vi "ThermalDiffusivity.vi"() -> ()   [LabVIEW 2014]
uses:
  Typedef_FindPortActions.ctl
  Typedef_TeachLabArduinos.ctl
  Typedef_DataLogger_Actions.ctl
  <vilib>/Utility/file.llb/Write To Spreadsheet File (DBL).vi
panel:
  out "Internal Temp vs Time":cluster{dbl[], dbl[]}(graph)
  out "External Temp":dbl format="%.2f"
  in  "Time Step (ms)":i32=500 min=5 max=5000 step=1
  out "Internal Temp":dbl format="%.2f"
  out "External Temp vs Time":cluster{dbl[], dbl[]}(graph)
  out "Elapsed Time (s)":dbl format="%.1f"
  in  "Filename Header":string="Data"
  in  "Maximum Log Time (s)":dbl=600.0 format="%#_6f"
  out "Status":enum16{"Logging", "Stopped"}(ring)=enum."Stopped"
  in  "Logging":cluster{"Start":bool, "Stop":bool}
  out "Last Save's Filename":string
  in  "Save Data":bool
  in  "Reset Graph":bool
  out "Error Out":errorcluster
  in  "Exit Program":bool
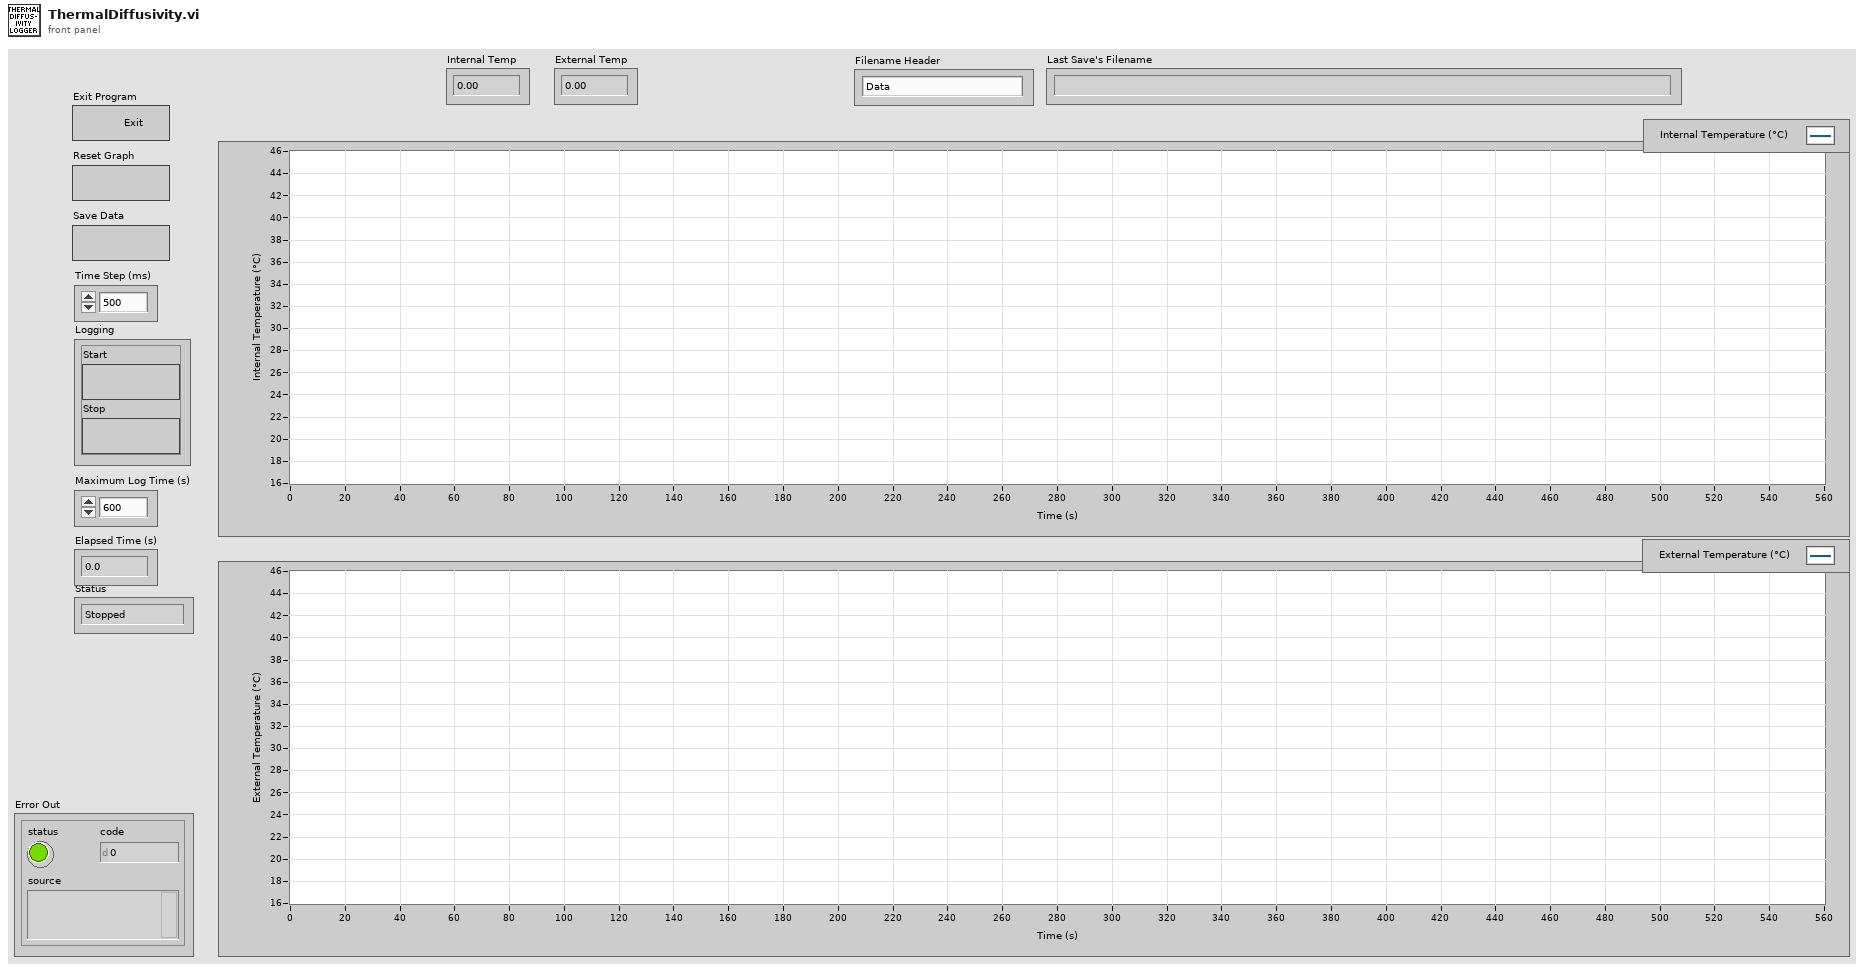
[diagram p1: front panel]
types:
  T1 = typedef "Typedef_FindPortActions.ctl" = enum16{"Reset List", "Find arduinos", "Get COM Port"}
  T2 = typedef "Typedef_TeachLabArduinos.ctl" = enum16{"FH", "AL", "CO", "TD"}
  T3 = typedef "Typedef_DataLogger_Actions.ctl" = enum16{"Connect", "Disconnect", "Get Reading", "Set Offset", "Get Offset", "Set Time Step", "Get Time Step", "Save Settings", "Disable Readings", "Enable Readings"}
  T4 = cluster{cluster{dbl[], dbl[]}, cluster{dbl[], dbl[]}}
  T5 = cluster{"Internal Temp":dbl, "External Temp":dbl}
  T6 = cluster{"Internal Temp vs Time In":cluster{"Array":dbl[], "Array":dbl[]}, "External Temp vs Time In":cluster{"Array":dbl[], "Array":dbl[]}}
  T7 = enum32{"invalid app kind", "Development System", "Run Time System", "Student Edition", "Embedded LabVIEW", "Evaluation", "Custom"}
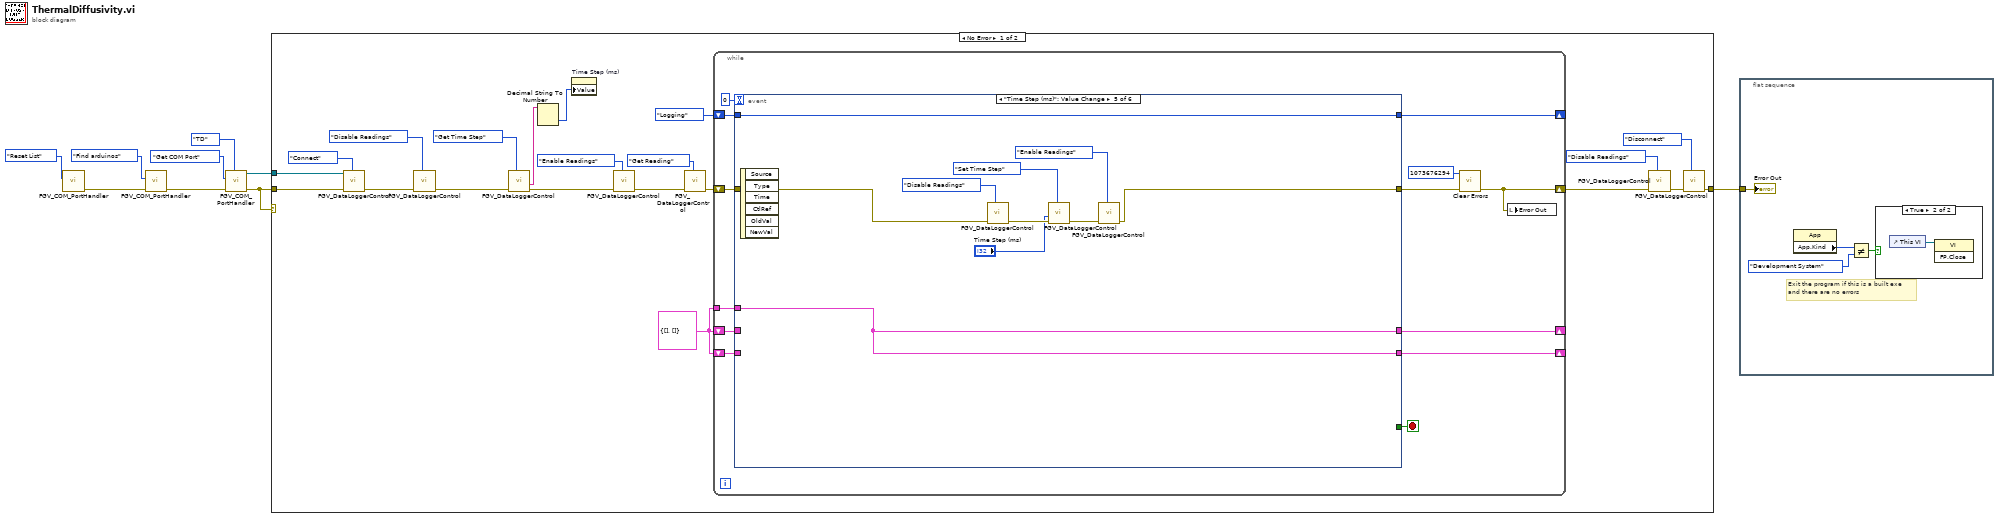
[diagram p0: block diagram]
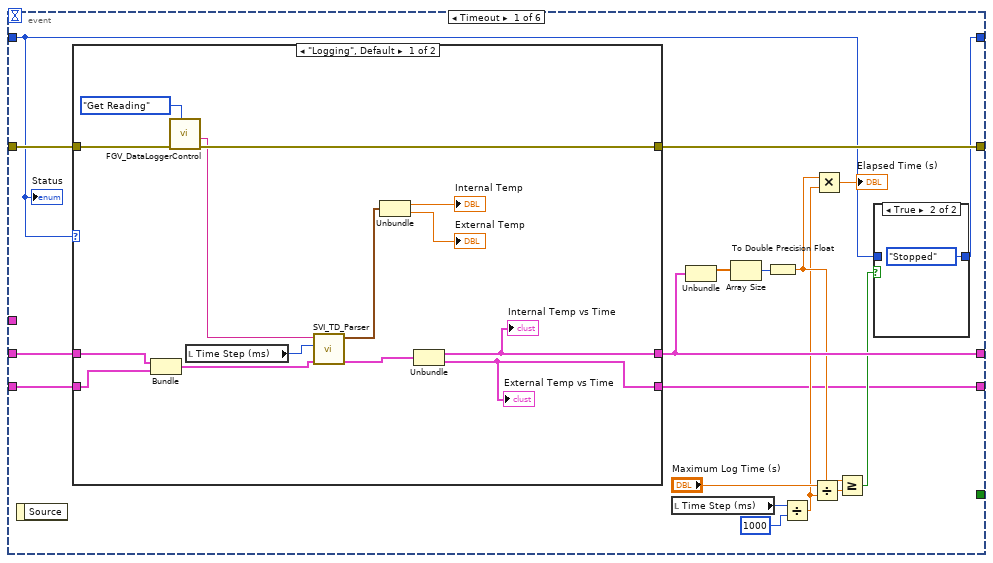
[diagram p3: hidden frame]
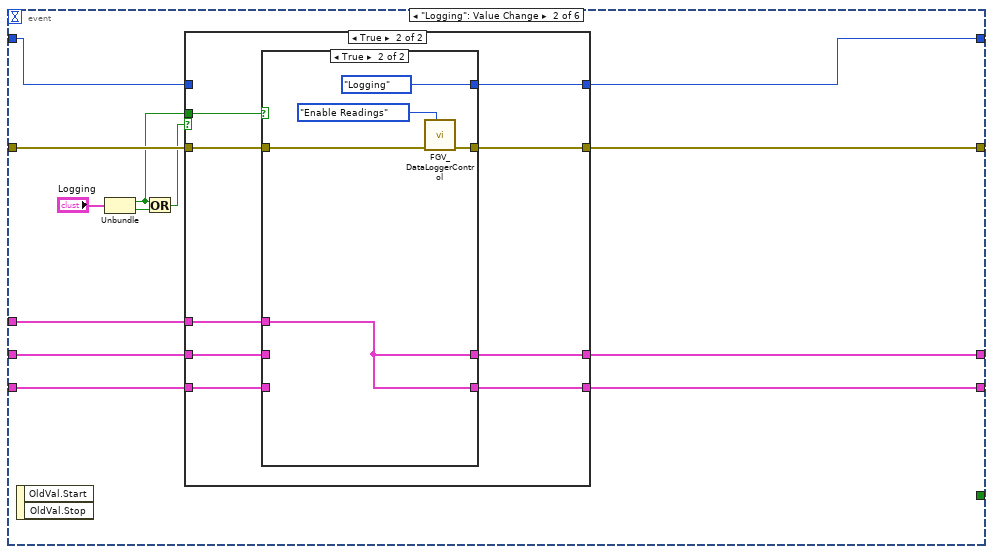
[diagram p6: hidden frame]
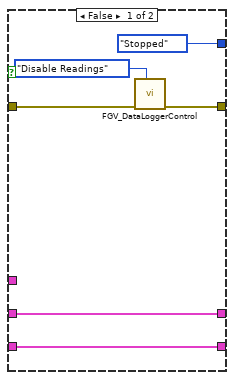
[diagram p8: hidden frame]
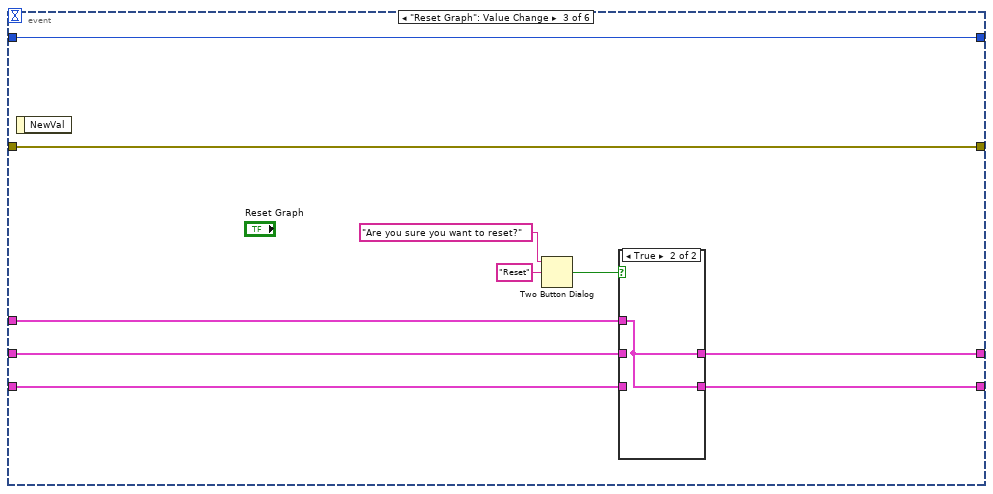
[diagram p9: hidden frame]
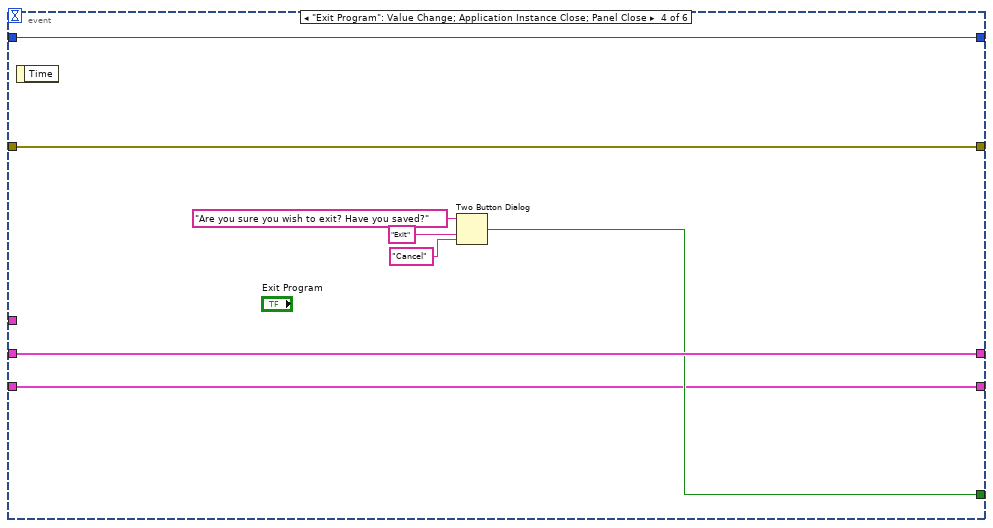
[diagram p11: hidden frame]
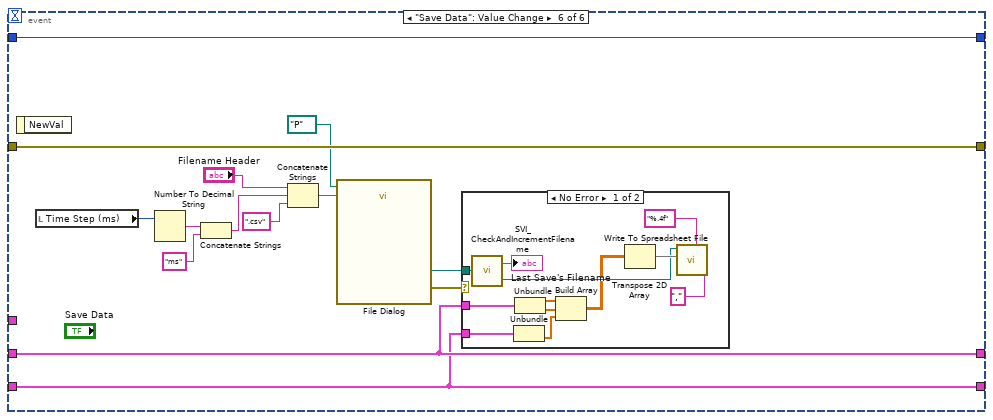
[diagram p12: hidden frame]
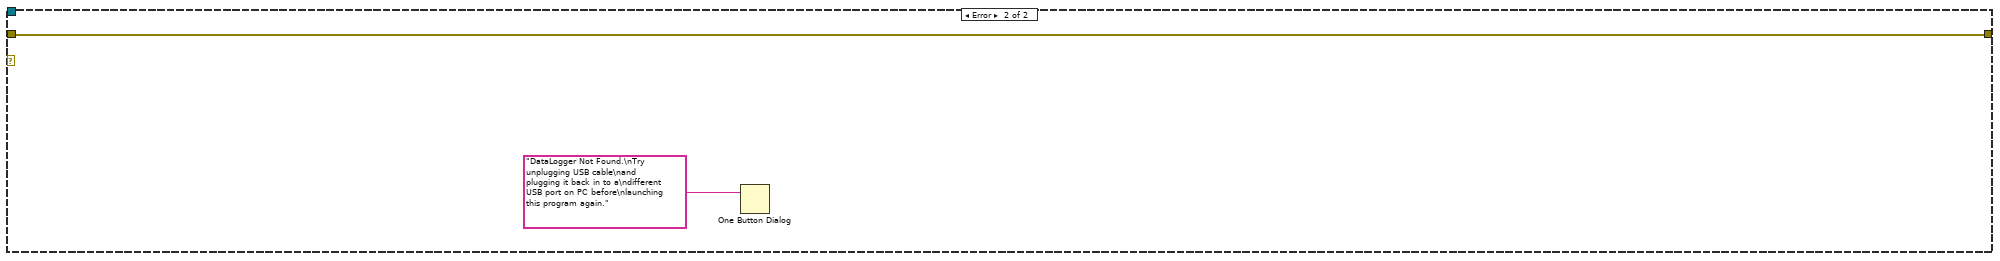
[diagram p14: hidden frame]
diagram:
  n1 = call "FGV_COM_PortHandler.vi"("Action"=Typedef_FindPortActions."Reset List") -> ("Error Out"=w5:errorcluster)  [unwired: 5 in, 2 out]
  n2 = call "FGV_COM_PortHandler.vi"("Error In"=w5, "Action"=Typedef_FindPortActions."Find arduinos") -> ("Error Out"=w9:errorcluster)  [unwired: 4 in, 2 out]
  n3 = call "FGV_COM_PortHandler.vi"("Device"=Typedef_TeachLabArduinos."TD", "Error In"=w9, "Action"=Typedef_FindPortActions."Get COM Port") -> ("Error Out"=w2:errorcluster, "COM Port"=w3:refnum<visa-resource-name>)  [unwired: 3 in, 1 out]
  n4 = case shown="No Error" w2 {
    tunnel: w2 -> [w29 w176]
    tunnel: w3 -> [w28 _]
    tunnel: [w25 w176] -> w1
    frame No Error {
      w10 = cluster{dbl[], dbl[]} {[], []}
      n5 = call "FGV_DataLoggerControl.vi"("Actions"=Typedef_DataLogger_Actions."Connect", "Error In"=w29, "VISA Refnum in"=w28) -> ("Error Out"=w21:errorcluster)  [unwired: 6 in, 2 out]
      n6 = call "FGV_DataLoggerControl.vi"("Actions"=Typedef_DataLogger_Actions."Disable Readings", "Error In"=w21) -> ("Error Out"=w20:errorcluster)  [unwired: 7 in, 2 out]
      n7 = call "FGV_DataLoggerControl.vi"("Actions"=Typedef_DataLogger_Actions."Get Time Step", "Error In"=w20) -> ("Error Out"=w18:errorcluster, "read buffer"=w24:string)  [unwired: 7 in, 1 out]
      n8 = Decimal String To Number(string=w24) -> (number=w23:i32)  [unwired: 2 in, 1 out]
      n9 = property on="Time Step (ms)" class="DigNum (strict)"("Value"=w23) -> ()  [unwired: 2 in, 2 out]
      n10 = call "FGV_DataLoggerControl.vi"("Actions"=Typedef_DataLogger_Actions."Enable Readings", "Error In"=w18) -> ("Error Out"=w11:errorcluster)  [unwired: 7 in, 2 out]
      n11 = call "FGV_DataLoggerControl.vi"("Actions"=Typedef_DataLogger_Actions."Get Reading", "Error In"=w11) -> ("Error Out"=w12:errorcluster)  [unwired: 7 in, 2 out]
      n12 = while {
        shift-right: [w40] -> _
        shift-left: w10 -> [w39]
        tunnel: w10 -> [w38]
        shift-right: [w36] -> _
        shift-left: enum16{"Logging", "Stopped"}."Logging" ("Status") -> [w37]
        shift-right: [w34] -> w16
        shift-left: w12 -> [w43]
        shift-right: [w31] -> _
        shift-left: w10 -> [w32]
        stop <- w42 stop-if-true
        n13 = event shown="[4] \"Time Step (ms)\": Value Change" {
          selector: _ -> [_ _ _ _ _ _]
          dyn-events: _ -> [_ _ _ _ _ _]
          timeout: 0 -> [_ _ _ _ _ _]
          tunnel: w43 -> [w61 w91 w127 w137 w142 w162]
          tunnel: [w60 w90 w127 w137 w143 w162] -> w33
          tunnel: [_ _ _ w133 _ _] -> w42
          tunnel: [w57 w84 w121 w138 w140 w150] -> w40
          tunnel: w39 -> [w59 w85 w119 w138 _ w150]
          tunnel: w38 -> [_ w83 w122 _ w140 _]
          tunnel: [w50 w93 w126 w132 w141 w154] -> w36
          tunnel: w37 -> [w49 w92 w126 w132 w141 w154]
          tunnel: w32 -> [w45 w81 w118 w131 _ w149]
          tunnel: [w44 w82 w120 w131 w140 w149] -> w31
          event Timeout {
            n14 = event-data() -> ()  [unwired: 1 in, 1 out]
            n15 = case shown="\"Logging\", Default" w49 {
              tunnel: w61 -> [w77 w79]
              tunnel: [w76 w79] -> w60
              tunnel: [w66 w80] -> w57
              tunnel: w59 -> [w71 w80]
              tunnel: w45 -> [w70 w78]
              tunnel: [w65 w78] -> w44
              frame "Logging", Default {
                n16 = Bundle(w71, w70) -> (w72:T4)  [unwired: 1 in]
                n17 = call "FGV_DataLoggerControl.vi"("Actions"=Typedef_DataLogger_Actions."Get Reading", "Error In"=w77) -> ("Error Out"=w76:errorcluster, "read buffer"=w74:string)  [unwired: 7 in, 1 out]
                n18 = local read "Time Step (ms)"() -> (w68:i32)
                n19 = call "SVI_TD_Parser.vi"("read buffer"=w74, "Time Step (ms)"=w68, "In"=w72) -> ("Current Values"=w67:T5, "Out"=w73:T6)  [unwired: 4 in]
                n20 = Unbundle(w67) -> ("Internal Temp"=→"Internal Temp":dbl, "External Temp"=→"External Temp":dbl)
                n21 = Unbundle(w73) -> ("Internal Temp vs Time In"=w66:cluster{"Array":dbl[], "Array":dbl[]}, "External Temp vs Time In"=w65:cluster{"Array":dbl[], "Array":dbl[]})
                "External Temp vs Time" <- w65
                "Internal Temp vs Time" <- w66
              }
              frame "Stopped" {
              }
            }
            n22 = local read "Time Step (ms)"() -> (w56:i32)
            n23 = Unbundle(w57) -> ("Array"=w58:dbl[])  [unwired: 1 out]
            n24 = Array Size(array=w58) -> (size(s)=w52:i32)
            n25 = To Double Precision Float(number=w52) -> (double precision float=w48:dbl)
            n26 = Divide(x=w56, y=1000) -> (x/y=w47:dbl)
            n27 = Divide(x="Maximum Log Time (s)", y=w47) -> (x/y=w53:dbl)
            n28 = Multiply(x=w48, y=w47) -> (x*y=→"Elapsed Time (s)":dbl)
            n29 = Greater Or Equal?(x=w48, y=w53) -> (x >= y?=w51:bool)
            n30 = case shown="True" w51 {
              tunnel: [w62 enum16{"Logging", "Stopped"}."Stopped" ("Status")] -> w50
              tunnel: w49 -> [w62 _]
              frame False {
              }
              frame True {
              }
            }
            "Status" <- w49
          }
          event "Logging": Value Change {
            n31 = event-data() -> ()  [unwired: 1 in, 2 out]
            n32 = Unbundle("Logging") -> ("Start"=w86:bool, "Stop"=w88:bool)
            n33 = Or(x=w86, y=w88) -> (x .or. y?=w87:bool)
            n34 = case shown="True" w87 {
              tunnel: [w97 w106] -> w93
              tunnel: w92 -> [w97 _]
              tunnel: w91 -> [w96 w105]
              tunnel: [w96 w104] -> w90
              tunnel: w86 -> [_ w103]
              tunnel: w85 -> [w95 w102]
              tunnel: [w95 w101] -> w84
              tunnel: w83 -> [_ w100]
              tunnel: [w94 w99] -> w82
              tunnel: w81 -> [w94 w98]
              frame False {
              }
              frame True {
                n35 = case shown="True" w103 {
                  tunnel: [enum16{"Logging", "Stopped"}."Stopped" ("Status") enum16{"Logging", "Stopped"}."Logging" ("Status")] -> w106
                  tunnel: w105 -> [w109 w115]
                  tunnel: [w110 w114] -> w104
                  tunnel: w102 -> [w108 _]
                  tunnel: [w108 w113] -> w101
                  tunnel: w100 -> [_ w113]
                  tunnel: [w107 w113] -> w99
                  tunnel: w98 -> [w107 _]
                  frame False {
                    n36 = call "FGV_DataLoggerControl.vi"("Actions"=Typedef_DataLogger_Actions."Disable Readings", "Error In"=w109) -> ("Error Out"=w110:errorcluster)  [unwired: 7 in, 2 out]
                  }
                  frame True {
                    n37 = call "FGV_DataLoggerControl.vi"("Actions"=Typedef_DataLogger_Actions."Enable Readings", "Error In"=w115) -> ("Error Out"=w114:errorcluster)  [unwired: 7 in, 2 out]
                  }
                }
              }
            }
          }
          event "Reset Graph": Value Change {
            n38 = event-data() -> ()  [unwired: 1 in, 1 out]
            n39 = Two Button Dialog(message="Are you sure you want to reset?", 2:"Reset" ("T button name (\"OK\")")) -> (T button?=w123:bool)  [unwired: 1 in]
            n40 = case shown="True" w123 {
              tunnel: w122 -> [_ w130]
              tunnel: [w129 w130] -> w121
              tunnel: [w128 w130] -> w120
              tunnel: w119 -> [w129 _]
              tunnel: w118 -> [w128 _]
              frame False {
              }
              frame True {
              }
            }
          }
          event "Exit Program": Value Change; Application Instance Close; Panel Close {
            n41 = event-data() -> ()  [unwired: 1 in, 1 out]
            n42 = Two Button Dialog(message="Are you sure you wish to exit? Have you saved?", 1:"Cancel" ("F button name (\"Cancel\")"), 2:"Exit" ("T button name (\"OK\")")) -> (T button?=w133:bool)
          }
          event "Time Step (ms)": Value Change {
            n43 = event-data() -> ()  [unwired: 1 in, 6 out]
            n44 = call "FGV_DataLoggerControl.vi"("Actions"=Typedef_DataLogger_Actions."Disable Readings", "Error In"=w142) -> ("Error Out"=w146:errorcluster)  [unwired: 7 in, 2 out]
            n45 = call "FGV_DataLoggerControl.vi"("Actions"=Typedef_DataLogger_Actions."Set Time Step", "Error In"=w146, "Value"="Time Step (ms)") -> ("Error Out"=w144:errorcluster)  [unwired: 6 in, 2 out]
            n46 = call "FGV_DataLoggerControl.vi"("Actions"=Typedef_DataLogger_Actions."Enable Readings", "Error In"=w144) -> ("Error Out"=w143:errorcluster)  [unwired: 7 in, 2 out]
          }
          event "Save Data": Value Change {
            n47 = event-data() -> ()  [unwired: 1 in, 1 out]
            n48 = local read "Time Step (ms)"() -> (w155:i32)
            n49 = Number To Decimal String(number=w155) -> (decimal integer string=w156:string)  [unwired: 1 in]
            n50 = Concatenate Strings(w156, "ms" ("string")) -> (w158:string)
            n51 = Concatenate Strings("Filename Header", w158, ".csv" ("default name")) -> (w160:string)
            n52 = call "File Dialog"("start path"=path "P:/", "default name"=w160) -> ("selected path"=w161:path, "error out"=w151:errorcluster)  [unwired: 10 in, 2 out]
            n53 = case shown="No Error" w151 {
              tunnel: w161 -> [w171 _]
              tunnel: w150 -> [w165 _]
              tunnel: w149 -> [w164 _]
              frame No Error {
                n54 = call "SVI_CheckAndIncrementFilename.vi"("selected path"=w171) -> ("Filename"=→"Last Save's Filename":string, "File Path"=w168:path)
                n55 = Unbundle(w164) -> (w163:dbl[])  [unwired: 1 out]
                n56 = Unbundle(w165) -> (w173:dbl[], w174:dbl[])
                n57 = Build Array(w173, w174, w163) -> (w167:dbl[][])
                n58 = Transpose 2D Array(2D array=w167) -> (transposed array=w169:dbl[][])
                n59 = call-poly <vilib>:"Write To Spreadsheet File.vi"("delimiter (\\t)"="," ("delimiter (\\t)"), "format (%.3f)"="%.4f", "2D data"=w169, "file path (dialog if empty)"=w168) -> ()  [unwired: 4 in, 1 out]
              }
              frame Error {
              }
            }
          }
        }
        n60 = call <vilib>:"Clear Errors.vi"("error in (no error)"=w33, "specific error code to clear (0: all)"=1073676294) -> ("error out"=w34:errorcluster)  [unwired: 4 in, 1 out]
        n61 = local write "Error Out"(w34) -> ()
      }
      n62 = call "FGV_DataLoggerControl.vi"("Actions"=Typedef_DataLogger_Actions."Disable Readings", "Error In"=w16) -> ("Error Out"=w15:errorcluster)  [unwired: 7 in, 2 out]
      n63 = call "FGV_DataLoggerControl.vi"("Actions"=Typedef_DataLogger_Actions."Disconnect", "Error In"=w15) -> ("Error Out"=w25:errorcluster)  [unwired: 7 in, 2 out]
    }
    frame Error {
      n64 = One Button Dialog(message="DataLogger Not Found.\nTry unplugging USB cable\nand plugging it back in to a\ndifferent USB port on PC before\nlaunching this program again.") -> ()  [unwired: 1 in, 1 out]
    }
  }
  n65 = flat-sequence {
    tunnel: w1 -> [w178]
    frame #0 {
      # "Exit the program if this is a built exe\nand there are no errors"
      n66 = property class="App"() -> ("App.Kind"=w179:T7)  [unwired: 2 in, 2 out]
      n67 = Not Equal?(x=w179, y=T7."Development System" ("Application:Kind 2")) -> (x != y?=w177:bool)
      n68 = case shown="True" w177 {
        frame False {
        }
        frame True {
          n69 = control-ref of="This VI"() -> (w181:refnum<vi>)
          n70 = invoke class="VI" method="FP.Close"(reference=w181) -> ()  [unwired: 2 in, 3 out]
        }
      }
      "Error Out" <- w178
    }
  }
